vi "超标留样全局.vi"() -> ()   [LabVIEW 2016, in "德润DR803F超标留样.lvlib"]
panel:
  in  "CODCr超标浓度":dbl
  in  "CODMn超标浓度":dbl
  in  "总氮超标浓度":dbl
  in  "总磷超标浓度":dbl
  in  "氨氮超标浓度":dbl
  out "仪器状态":T1 {"门状态" items=["关闭", "打开"]; "采样模式" items=["定时留样"=1, "时间等比"=2, "同步留样"=3, "外控留样"=4, "超标留样"=5]; "工作进程" items=["清洗管路初始化", "采样瓶位置初始化", "采样瓶排空", "清洗管下降", "采样瓶清洗", "清洗管上升", "外置泵延时", "管路润洗", "进样1", "进样2", "排空管路", "采样瓶位置调整", "待机"]; "仪器时间" format="%<%Y/%m/%d %H:%M:%S>T"; "工作状态" items=["停止", "运行"]}
  out "超标留样等待时间/s":dbl
  out "流程中":bool
  out "超标留样信号":bool
  out "通讯":bool
  in  "VISA resource name":refnum<visa-resource-name>="COM2" caption="VISA资源名称"
  in  "外控留样读取更新":bool
  out "外控留样":T2
  in  "读取更新":bool
  out "超标留样":T3={"当前瓶号："=0.0, "平行样："=0.0, "留样瓶数："=0.0, "每瓶次数："=0.0, "每次留样："=0.0, "时间间隔："=0.0, "COD联机："=2, "氨氮联机："=2, "4mA浓度："=0.0, "20mA浓度："=0.0, "超标浓度："=0.0, "4mA浓度："=0.0, "20mA浓度:"=0.0, "超标浓度："=0.0} {"COD联机：" items=["继电器"=1, "模拟输入"=2, "串口连接"=3]; "氨氮联机：" items=["继电器"=1, "模拟输入"=2, "串口连接"=3]}
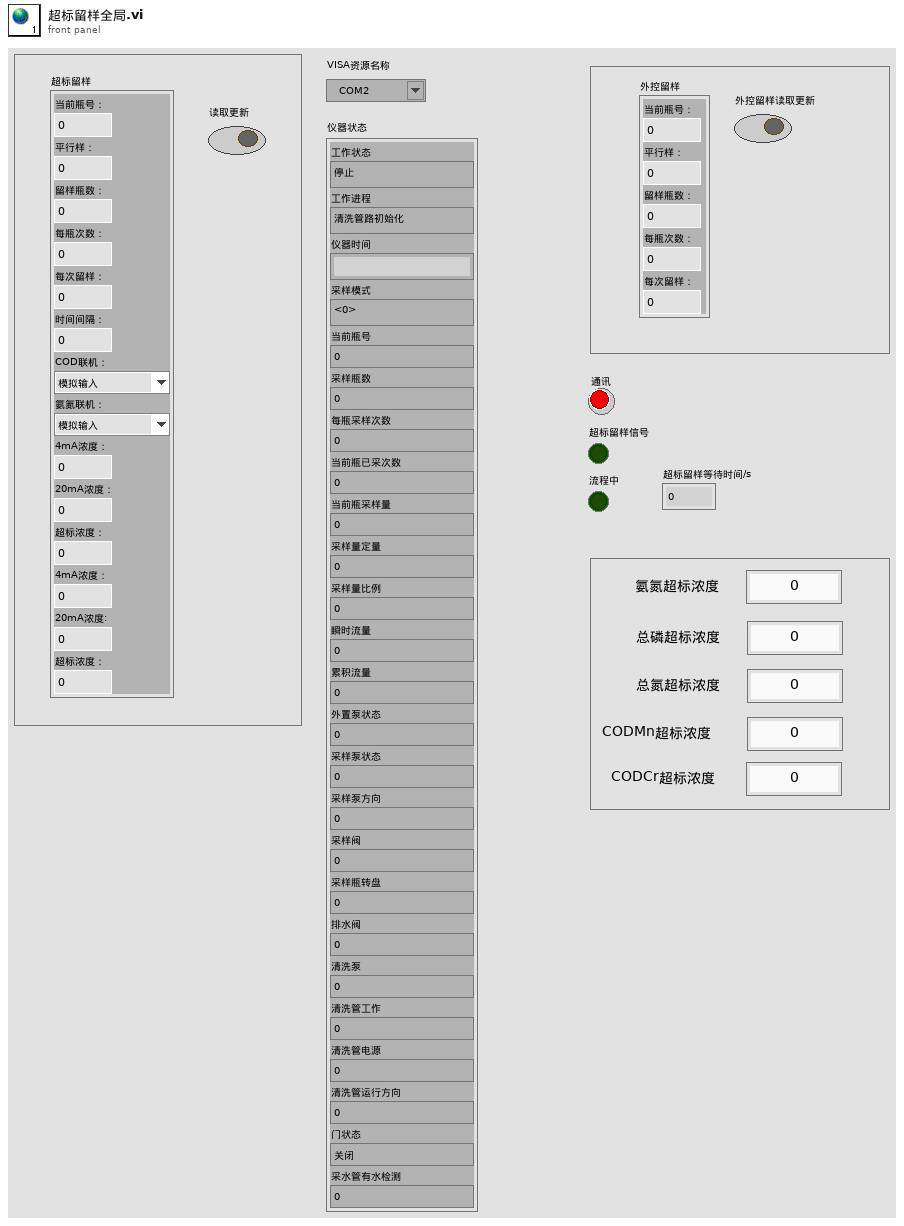
[diagram p1: front panel]
types:
  T1 = cluster{"工作状态":u16, "工作进程":u16, "仪器时间":timestamp, "采样模式":u16, "当前瓶号":dbl, "采样瓶数":dbl, "每瓶采样次数":dbl, "当前瓶已采次数":dbl, "当前瓶采样量":dbl, "采样量定量":dbl, "采样量比例":dbl, "瞬时流量":dbl, "累积流量":dbl, "外置泵状态":dbl, "采样泵状态":dbl, "采样泵方向":dbl, "采样阀":dbl, "采样瓶转盘":dbl, "排水阀":dbl, "清洗泵":dbl, "清洗管工作":dbl, "清洗管电源":dbl, "清洗管运行方向":dbl, "门状态":u16, "采水管有水检测":dbl}
  T2 = cluster{"当前瓶号：":dbl, "平行样：":dbl, "留样瓶数：":dbl, "每瓶次数：":dbl, "每次留样：":dbl}
  T3 = cluster{"当前瓶号：":dbl, "平行样：":dbl, "留样瓶数：":dbl, "每瓶次数：":dbl, "每次留样：":dbl, "时间间隔：":dbl, "COD联机：":u16, "氨氮联机：":u16, "4mA浓度：":dbl, "20mA浓度：":dbl, "超标浓度：":dbl, "4mA浓度：":dbl, "20mA浓度:":dbl, "超标浓度：":dbl}
diagram:
